vi "DllFxpConvertTemp.vi"(6 "ready for output":bool, 9 "input valid":bool, 11 "x":fxp<+/-,16,1>) -> (1 "output valid":bool, 2 "overflow?":bool, 3 "y":fxp<+/-,16,1> format="%.16g", 4 "ready for input":bool)   [LabVIEW 2017]
uses:
  <vilib>/rvi/FXPMathLib/FxpConvert/subVIs/nifxpmath_Convert_SimConfig.ctl
  <vilib>/fxp/LVFixedPointQuantizationPolicyTypeDef.ctl
  <vilib>/fxp/LVFixedPointOverflowPolicyTypeDef.ctl
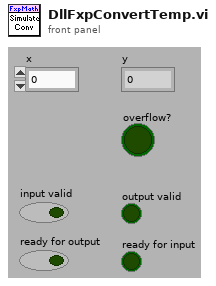
[diagram p1: front panel]
types:
  T1 = typedef "nifxpmath_Convert_SimConfig.ctl" = cluster{"kXSigned":bool, "kXWl":u32, "kXIwl":i32, "kYSigned":bool, "kYWl":u32, "kYIwl":i32, "Fixed-Point:Quantization Policy":T2, "Fixed-Point:Overflow Policy":T3, "OutputRegister":bool, "SupportSCTL?":bool}
  T2 = typedef "LVFixedPointQuantizationPolicyTypeDef.ctl" = enum32{"Truncate", "Round-Half-Up (Asymmetric)", "Round-Half-Even"}
  T3 = typedef "LVFixedPointOverflowPolicyTypeDef.ctl" = enum32{"Wrap", "Saturate"}
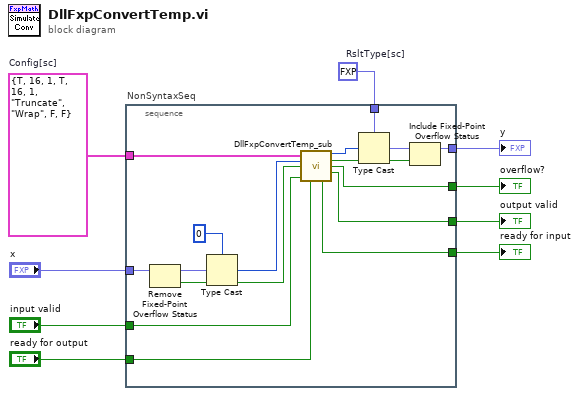
[diagram p0: block diagram]
diagram:
  w1 = T1 {"kXSigned"=TRUE, "kXWl"=16, "kXIwl"=1, "kYSigned"=TRUE, "kYWl"=16, "kYIwl"=1, "Fixed-Point:Quantization Policy"=enum."Truncate", "Fixed-Point:Overflow Policy"=enum."Wrap", "OutputRegister"=FALSE, "SupportSCTL?"=FALSE}  # Config[sc]
  w6 = fxp<+/-,16,1> 0.0  # RsltType[sc]
  n1 = stacked-sequence "NonSyntaxSeq" {
    tunnel: "x" -> [w16]
    tunnel: w6 -> [w25]
    tunnel: [w13] -> w5
    tunnel: "input valid" -> [w22]
    tunnel: [w10] -> w4
    tunnel: [w18] -> w2
    tunnel: [w17] -> w3
    tunnel: "ready for output" -> [w20]
    tunnel: w1 -> [w19]
    frame #0 {
      n2 = Remove Fixed-Point Overflow Status(3:w16) -> (0:w12:bool, 1:w15:fxp<+/-,16,1>)
      n3 = Type Cast(type=u64 0, x=w15) -> (*(type *) &x=w23:u64)
      n4 = call <vilib>:"DllFxpConvertTemp_sub.vi"("Config[sc]"=w19, "x"=w23, "x ovfl status"=w12, "input valid"=w22, "ready for output"=w20) -> ("y"=w21:u64, "y ovfl status"=w11:bool, "operational overflow"=w10:bool, "output valid"=w17:bool, "ready for input"=w18:bool)  [unwired: 2 in, 4 out]
      n5 = Type Cast(type=w25, x=w21) -> (*(type *) &x=w14:fxp<+/-,16,1>)
      n6 = Include Fixed-Point Overflow Status(2:w11, 3:w14) -> (1:w13:fxp<+/-,16,1>)
    }
  }
  "overflow?" <- w4
  "y" <- w5
  "output valid" <- w3
  "ready for input" <- w2
